vi "gerenciador_erro.vi"(8 "error in":errorcluster, 11 "Estado in":T1) -> (0 "error out":errorcluster, 3 "States":T1)   [LabVIEW 2018]
uses:
  Controls/SM-SG State.ctl
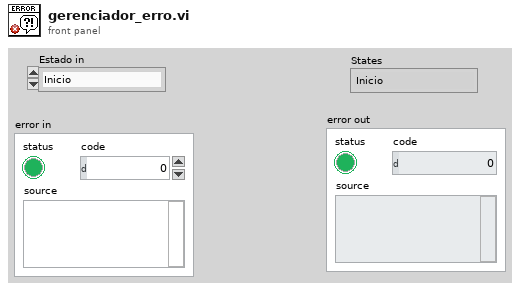
[diagram p1: front panel]
types:
  T1 = typedef "SM-SG State.ctl" = enum16{"Inicio", "Aguarda Evento", "Desenha Onda", "Mostra Sinal", "Limpa Gráfico", "Adicionar", "Remover", "Salvar", "Carregar", "Gera onda", "Valida onda", "Parar geração", "Gerenciador Erro", "Ajuda", "Sobre", "Sair"}
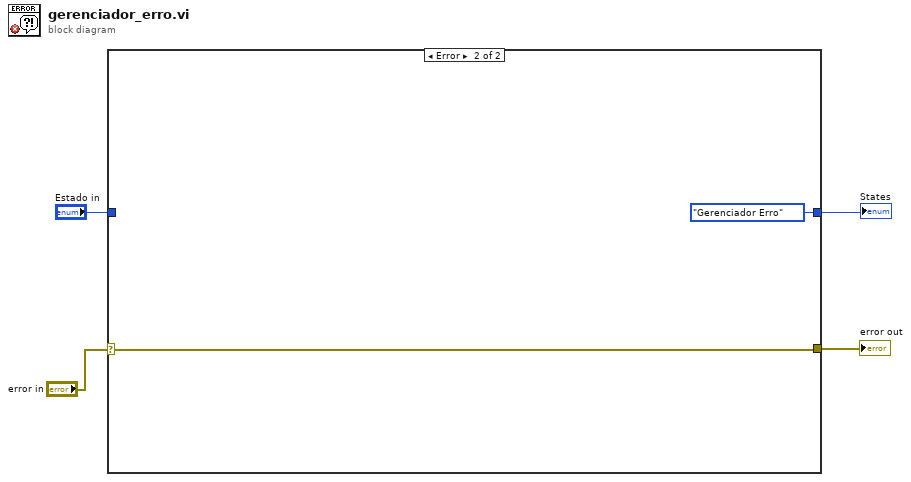
[diagram p0: block diagram]
diagram:
  n1 = case shown="Error" "error in" {
    selector: "error in" -> [w6 w8]
    tunnel: [w6 w8] -> w3
    tunnel: [w5 SM-SG_State."Gerenciador Erro" ("Estado in")] -> w1
    tunnel: "Estado in" -> [w5 _]
    frame No Error {
      # "Estado sem erro: Mesmo 'Próximo estado' é passado para o programa."
    }
    frame Error {
    }
  }
  "error out" <- w3
  "States" <- w1
